vi "Auton Edit Queue.vi"   [LabVIEW 2017]
uses:
  Robot Global Data.vi
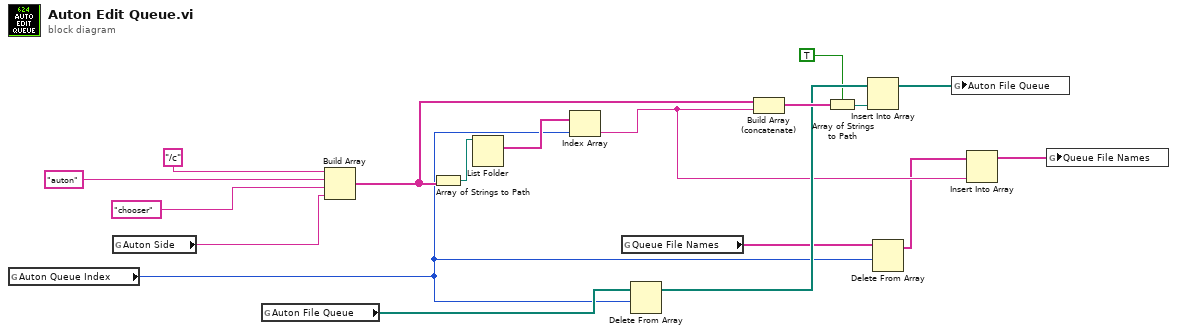
[diagram p0: block diagram]
diagram:
  n1 = global read "Robot Global Data.vi" "Auton Queue Index"() -> (w7:i32)
  n2 = global read "Robot Global Data.vi" "Auton Side"() -> (w11:string)
  n3 = global read "Robot Global Data.vi" "Auton File Queue"() -> (w9:path[])
  n4 = Build Array("/c", "auton", "chooser" ("element"), w11) -> (w17:string[])
  n5 = Array of Strings to Path(0:w17) -> (2:w16:path)  [unwired: 1 in]
  n6 = List Folder(path=w16) -> (filenames=w10:string[])  [unwired: 3 in, 3 out]
  n7 = Index Array(array=w10, index=w7) -> (element=w5:string)
  n8 = global read "Robot Global Data.vi" "Queue File Names"() -> (w6:string[])
  n9 = Delete From Array(array=w9, length=w7) -> (array with subset deleted=w8:path[])  [unwired: 1 in, 1 out]
  n10 = Build Array (concatenate)(w17, w5) -> (w18:string[])
  n11 = Array of Strings to Path(0:w18, 1:TRUE) -> (2:w12:path)
  n12 = Insert Into Array(array=w8, new element=w12) -> (w2:path[])  [unwired: 1 in]
  n13 = Delete From Array(array=w6, length=w7) -> (array with subset deleted=w4:string[])  [unwired: 1 in, 1 out]
  n14 = global write "Robot Global Data.vi" "Auton File Queue"(w2) -> ()
  n15 = Insert Into Array(array=w4, new element=w5) -> (w3:string[])  [unwired: 1 in]
  n16 = global write "Robot Global Data.vi" "Queue File Names"(w3) -> ()
